vi "UpdateButtons.vi"(10 "Currency":T1, 11 "Array":refnum<vi>[](array[refnum])) -> (3 "Values Array":dbl[](array[numeric]))   [LabVIEW 2020]
uses:
  Controls/Currency Enum.ctl
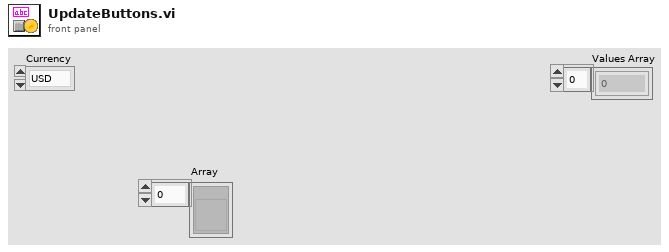
[diagram p1: front panel]
types:
  T1 = typedef "Currency Enum.ctl" = enum16{"USD", "MXN", "EUR"}
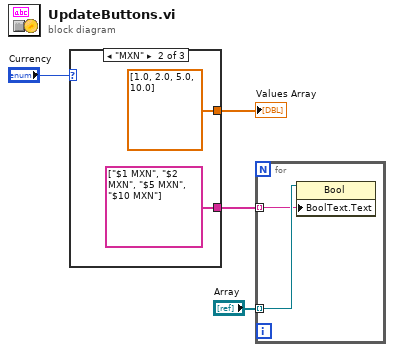
[diagram p0: block diagram]
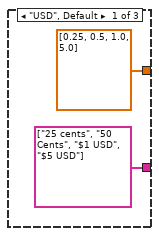
[diagram p2: hidden frame]
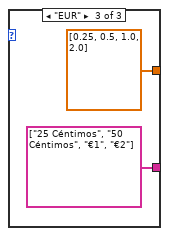
[diagram p3: hidden frame]
diagram:
  n1 = case shown="\"MXN\"" "Currency" {
    tunnel: [string[] ["25 cents", "50 Cents", "$1 USD", "$5 USD"] string[] ["$1 MXN", "$2 MXN", "$5 MXN", "$10 MXN"] string[] ["25 Céntimos", "50 Céntimos", "€1", "€2"]] -> w2
    tunnel: [dbl[] [0.25, 0.5, 1.0, 5.0] dbl[] [1.0, 2.0, 5.0, 10.0] dbl[] [0.25, 0.5, 1.0, 2.0]] -> w1
    frame "USD", Default {
    }
    frame "MXN" {
    }
    frame "EUR" {
    }
  }
  "Values Array" <- w1
  n2 = for {
    tunnel: "Array" -> [w12] mode=indexing
    tunnel: w2 -> [w11] mode=indexing
    n3 = property class="Bool"(reference=w12, "BoolText.Text"=w11) -> ()  [unwired: 1 in, 2 out]
  }
